vi "Calculate Statistics.vi"(8 "error in (no error)":errorcluster, 11 "Pips in":refnum<class "Pips.lvclass">) -> (0 "error out":errorcluster, 2 "Coverage Statistics":T1 {"TestCases.BlockedPct" format="%.1g"; "TestCases.SkippedPct" format="%.1g"; "TestCases.FailedPct" format="%.1g"; "TestCases.NotImplementedPct" format="%.1g"; "TestCases.ImplementedPct" format="%.1g"; "TestCases.PassPct" format="%.1g"; "TestCases.FullyCoveredPct" format="%.1g"; "Requirements.NotCoveredPct" format="%.1g"; "Requirements.PartiallyCoveredPct" format="%.1g"; "Requirements.FullyCoveredPct" format="%.1g"}, 3 "Pips out":refnum<class "Pips.lvclass">)   [LabVIEW 2021, in "Bananas.lvlib" / "Pips.lvclass"]
uses:
  Pips.lvclass
  statistics -- cluster.ctl
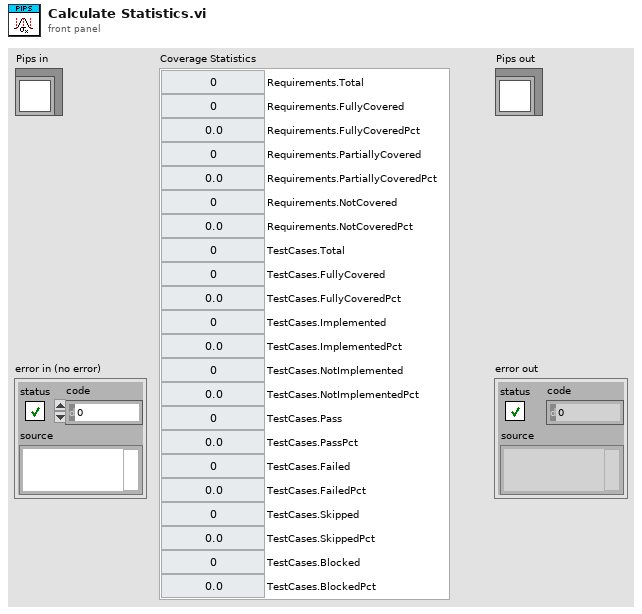
[diagram p1: front panel]
types:
  T1 = typedef "Bananas.lvlib/Pips.lvclass/statistics -- cluster.ctl" = cluster{"Requirements.Total":u32, "Requirements.FullyCovered":u32, "Requirements.FullyCoveredPct":dbl, "Requirements.PartiallyCovered":u32, "Requirements.PartiallyCoveredPct":dbl, "Requirements.NotCovered":u32, "Requirements.NotCoveredPct":dbl, "TestCases.Total":u32, "TestCases.FullyCovered":u32, "TestCases.FullyCoveredPct":dbl, "TestCases.Implemented":u32, "TestCases.ImplementedPct":dbl, "TestCases.NotImplemented":u32, "TestCases.NotImplementedPct":dbl, "TestCases.Pass":u32, "TestCases.PassPct":dbl, "TestCases.Failed":u32, "TestCases.FailedPct":dbl, "TestCases.Skipped":u32, "TestCases.SkippedPct":dbl, "TestCases.Blocked":u32, "TestCases.BlockedPct":dbl}
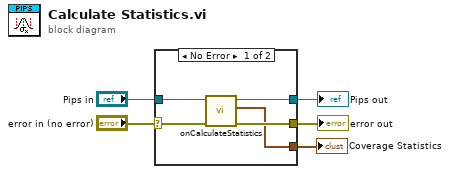
[diagram p0: block diagram]
diagram:
  n1 = case shown="No Error" "error in (no error)" {
    selector: "error in (no error)" -> [w8 w12]
    tunnel: [w7 w12] -> w4
    tunnel: [w10 w11] -> w2
    tunnel: "Pips in" -> [w9 w11]
    tunnel: [w6 _] -> w1
    frame No Error {
      n2 = call-dynamic "onCalculateStatistics.vi"("error in (no error)"=w8, "Pips in"=w9) -> ("error out"=w7:errorcluster, "Coverage Statistics"=w6:T1, "Pips out"=w10:refnum<class "Pips.lvclass">)  [unwired: 7 in]
    }
    frame Error {
    }
  }
  "error out" <- w4
  "Pips out" <- w2
  "Coverage Statistics" <- w1
